vi "Create Subscription.vi"(5 "Inbound Ack":refnum<user-event>, 7 "Inbound Message":refnum<user-event>, 8 "error in (no error)":errorcluster, 9 "SessionMailbox":refnum<queue>, 10 "QoS":T1, 11 "Topic Filter":string) -> (0 "error out":errorcluster, 3 "Subscription out":refnum<class "_Subscription.lvclass">)   [LabVIEW 2013, in "MQTT Server.lvlib" / "_Subscription.lvclass"]
uses:
  _Subscription.lvclass
  <vilib>/LabVIEW Open Source Project/MQTT Control Packets/Control Packets/ControlPacket/QualityOfService -- enum.ctl
  <vilib>/LabVIEW Open Source Project/MQTT Connection/MQTT_Base/Base Class/Response -- cluster.ctl
  <vilib>/LabVIEW Open Source Project/MQTT Control Packets/Control Packets/ControlPacket/ControlPacket.lvclass
  <vilib>/LabVIEW Open Source Project/MQTT Control Packets/Control Packets/PUBLISH/PUBLISH.lvclass
  <vilib>/LabVIEW Open Source Project/MQTT Control Packets/Control Packets/Ack/Ack.lvclass
  Queued Message -- cluster.ctl
  _Subscription.lvclass/_Subscription.ctl
  TopicFilter/_TopicFilter.lvclass
  <vilib>/LabVIEW Open Source Project/MQTT Connection/MQTT_Base/Base Class/MQTT_Base.lvclass
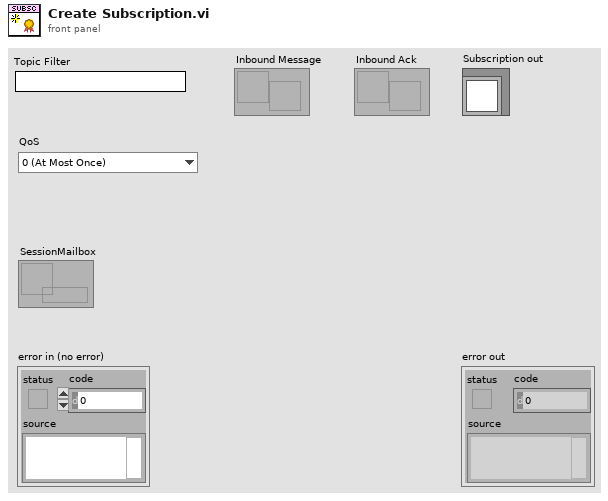
[diagram p1: front panel]
types:
  T1 = typedef "MQTT_Control_Packets.lvlib/ControlPacket.lvclass/QualityOfService -- enum.ctl" = enum16{"0 (At Most Once)", "1 (At Least Once)", "2 (Exactly Once)"}
  T2 = typedef "MQTT Server.lvlib/_Subscription.lvclass/Queued Message -- cluster.ctl" = cluster{"Message":refnum<class "PUBLISH.lvclass">, "PUBREC received":bool}
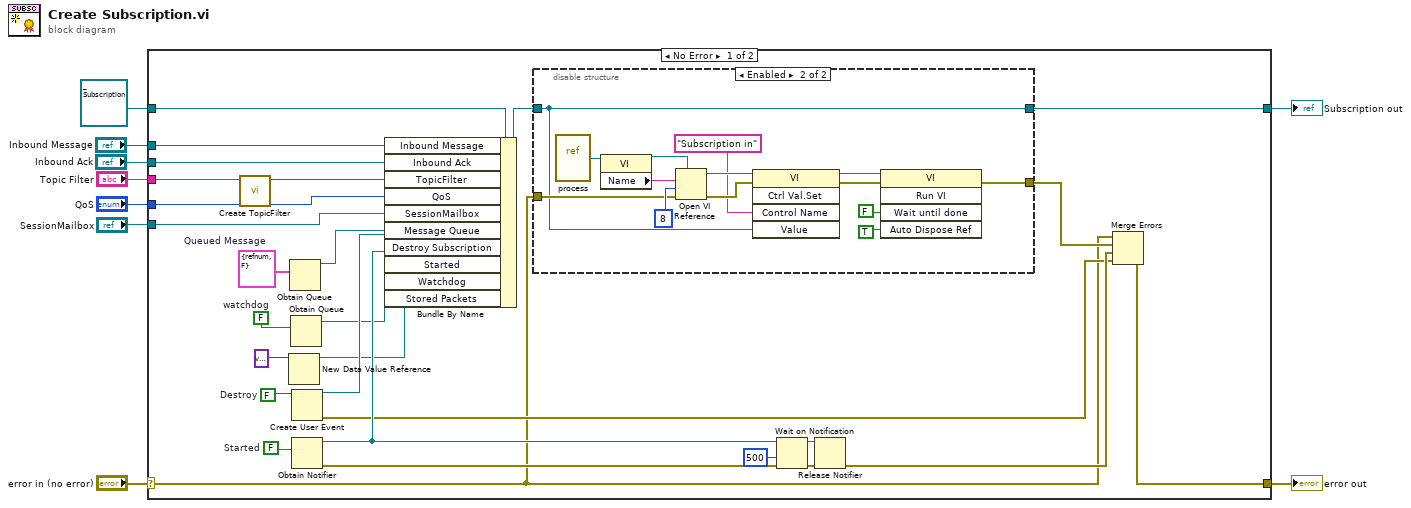
[diagram p0: block diagram]
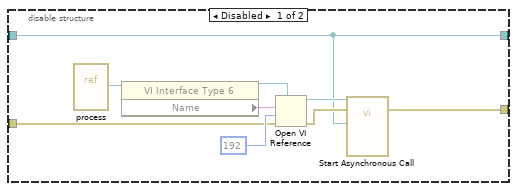
[diagram p2: hidden frame]
diagram:
  n1 = case shown="No Error" "error in (no error)" {
    selector: "error in (no error)" -> [w15 w62]
    tunnel: [w24 w62] -> w8
    tunnel: [w16 w61] -> w6
    tunnel: refnum<class "_Subscription.lvclass"> refnum ("Subscription in") -> [w35 w61]
    tunnel: "Topic Filter" -> [w23 _]
    tunnel: "QoS" -> [w37 _]
    tunnel: "SessionMailbox" -> [w36 _]
    tunnel: "Inbound Message" -> [w33 _]
    tunnel: "Inbound Ack" -> [w12 _]
    frame No Error {
      w14 = FALSE  # watchdog
      w21 = FALSE  # Destroy
      w32 = FALSE  # Started
      w34 = T2 {"Message"=refnum, "PUBREC received"=FALSE}  # Queued Message
      n2 = call "Create TopicFilter.vi"("Topic Filter"=w23) -> ("TopicFilter out"=w22:refnum<class "_TopicFilter.lvclass">)  [unwired: 9 in, 1 out]
      n3 = New Data Value Reference(data value=variant ("Stored Packets")) -> (data value reference=w10:refnum<data-value>)  [unwired: 1 in, 1 out]
      n4 = Obtain Queue(element data type=w34) -> (queue out=w31:refnum<queue>)  [unwired: 4 in, 2 out]
      n5 = Obtain Queue(element data type=w14) -> (queue out=w13:refnum<queue>)  [unwired: 4 in, 2 out]
      n6 = Create User Event(user event datatype=w21) -> (user event=w20:refnum<user-event>, error out=w19:errorcluster)  [unwired: 1 in]
      n7 = Obtain Notifier(notification data type=w32) -> (notifier out=w30:refnum<notifier>, error out=w27:errorcluster)  [unwired: 3 in, 1 out]
      n8 = Bundle By Name(cluster=w35, "Inbound Message"=w33, "Inbound Ack"=w12, "TopicFilter"=w22, "QoS"=w37, "SessionMailbox"=w36, "Message Queue"=w31, "Destroy Subscription"=w20, "Started"=w30, "Watchdog"=w13, "Stored Packets"=w10) -> (w17:refnum<class "_Subscription.lvclass">)
      n9 = disable-structure shown="Enabled" {
        disable-tunnel: w15 -> [w41 w57]
        disable-tunnel: w17 -> [w39 w50]
        disable-tunnel: [w40 w54] -> w18
        disable-tunnel: [w39 w50] -> w16
        frame Disabled {
          n10 = vi-ref "process.vi"() -> (w38:refnum<vi>)
          n11 = property class="VI Interface Type 6"(reference=w38) -> (reference out=w45:refnum<vi>, "Name"=w46:string)  [unwired: 1 in, 1 out]
          n12 = Open VI Reference(type specifier VI Refnum (for type only)=w45, vi path=w46, options=192, error in (no error)=w41) -> (vi reference=w44:refnum<vi>, error out=w43:errorcluster)  [unwired: 2 in]
          n13 = call-by-ref "Start Asynchronous Call"(reference=w44, error in=w43, "Subscription in"=w39) -> (error out=w40:errorcluster)  [unwired: 11 in, 1 out]
        }
        frame Enabled {
          n14 = vi-ref "process.vi"() -> (w47:refnum<vi>)
          n15 = property class="VI"(reference=w47) -> (reference out=w59:refnum<vi>, "Name"=w60:string)  [unwired: 1 in, 1 out]
          n16 = Open VI Reference(type specifier VI Refnum (for type only)=w59, vi path=w60, options=8, error in (no error)=w57) -> (vi reference=w52:refnum<vi>, error out=w53:errorcluster)  [unwired: 2 in]
          n17 = invoke class="VI" method="Ctrl Val.Set"(reference=w52, error in=w53, "Control Name"="Subscription in", "Value"=w50) -> (reference out=w49:refnum<vi>, error out=w48:errorcluster)  [unwired: 1 in, 3 out]
          n18 = invoke class="VI" method="Run VI"(reference=w49, error in=w48, "Wait until done"=FALSE ("Wait Until Done"), "Auto Dispose Ref"=TRUE ("Auto Dispose Reference")) -> (error out=w54:errorcluster)  [unwired: 1 in, 4 out]
        }
      }
      n19 = Wait on Notification(notifier=w30, timeout in ms (-1)=500, error in (no error)=w27) -> (notifier out=w28:refnum<notifier>, error out=w26:errorcluster)  [unwired: 1 in, 2 out]
      n20 = Release Notifier(notifier=w28, error in (no error)=w26) -> (error out=w25:errorcluster)  [unwired: 1 in, 2 out]
      n21 = Merge Errors(w15, w18, w25, w19) -> (w24:errorcluster)
    }
    frame Error {
    }
  }
  "error out" <- w8
  "Subscription out" <- w6
